vi "Notebook Content Storage.vi"(6 "Save(T)/Load(F)":bool, 8 "Error In":errorcluster, 10 "path":path, 11 ".NET Refnum in":refnum<k24>) -> (0 "Error Out":errorcluster, 3 "RTF content":string)   [LabVIEW 2019, in "Notebook.lvlib"]
uses:
  Notebook.lvlib
  System.Windows.Forms
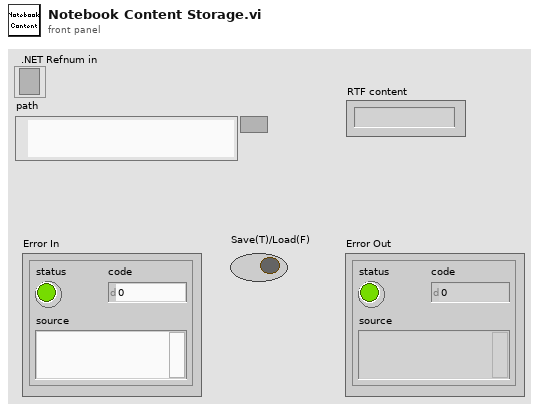
[diagram p1: front panel]
types:
  T1 = enum16{"open", "replace", "create", "open or create", "replace or create", "replace or create with confirmation"}
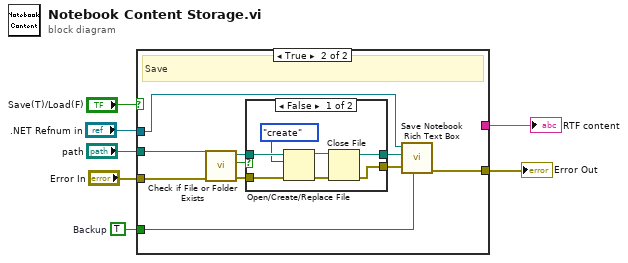
[diagram p0: block diagram]
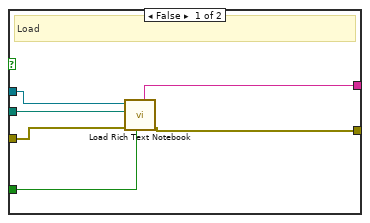
[diagram p2: hidden frame]
diagram:
  w2 = TRUE  # Backup
  n1 = case shown="True" "Save(T)/Load(F)" {
    tunnel: ".NET Refnum in" -> [w12 w18]
    tunnel: "Error In" -> [w11 w17]
    tunnel: [w10 w16] -> w5
    tunnel: "path" -> [w13 w15]
    tunnel: w2 -> [w9 w14]
    tunnel: [w8 _] -> w1
    frame False {
      # "Load"
      n2 = call "Load Rich Text Notebook.vi"("Backup?"=w9, "Error In"=w11, "File Path Control"=w13, ".NET Refnum in"=w12) -> ("Error Out"=w10:errorcluster, "RTF content"=w8:string)  [unwired: 3 in, 3 out]
    }
    frame True {
      # "Save"
      n3 = call <vilib>:"Check if File or Folder Exists.vi"("error in (no error)"=w17, "path"=w15) -> ("error out"=w19:errorcluster, "file or folder exists?"=w21:bool, "dup path"=w20:path)  [unwired: 7 in]
      n4 = case shown="False" w21 {
        tunnel: w20 -> [w30 w32]
        tunnel: [w24 w32] -> w23
        tunnel: w19 -> [w28 w31]
        tunnel: [w26 w31] -> w22
        frame False {
          n5 = Open/Create/Replace File(file path (use dialog)=w30, error in=w28, operation (0:open)=T1."create") -> (refnum out=w25:refnum<file>, error out=w27:errorcluster)  [unwired: 3 in, 1 out]
          n6 = Close File(refnum=w25, error in=w27) -> (path=w24:path, error out=w26:errorcluster)
        }
        frame True {
        }
      }
      n7 = call "Save Notebook Rich Text Box.vi"("Backup?"=w14, "Error In"=w22, "File Path Control"=w23, ".NET Refnum in"=w18) -> ("Error Out"=w16:errorcluster)  [unwired: 5 in, 2 out]
    }
  }
  "Error Out" <- w5
  "RTF content" <- w1
